vi "onStart.vi"(8 "error in (no error)":errorcluster, 11 "DAQmx":refnum<class "DAQmx.lvclass">) -> (0 "error out":errorcluster, 3 "DAQmx out":refnum<class "DAQmx.lvclass">)   [LabVIEW 2016, in "DAQmx.lvclass"]
doc: "JKI State Machine Objects (SMO) 1.2.1.55\nJKI - JKI\nCopyright (c) 2017, JKI"
uses:
  DAQmx.lvclass
  DAQ/DAQ.lvclass
panel:
  # "For instructions on how to use the JKI State Machine Objects, examples and video tutorials, visit:\nhttp://jki.net/state-machine-objects/\n\nJKI State Machine Objects™\nhttp://jki.net/state-machine-objects/\nCopyright (C) 2005-2015, JKI <info@jki.net>\nALL RIGHTS RESERVED"
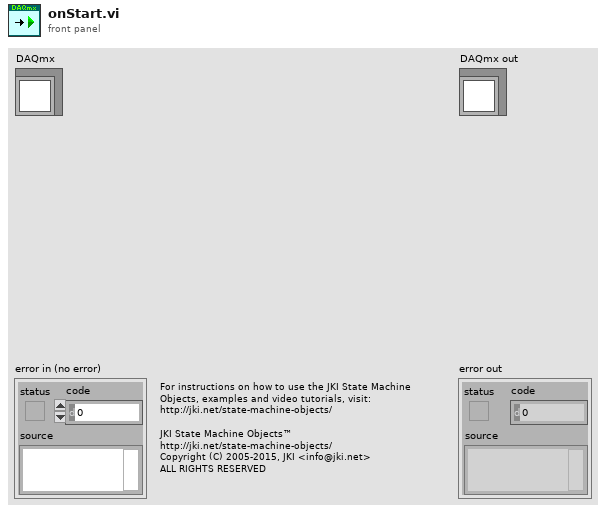
[diagram p1: front panel]
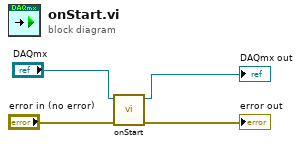
[diagram p0: block diagram]
diagram:
  n1 = call-parent "onStart.vi"("error in (no error)"="error in (no error)", "DAQ"="DAQmx") -> ("error out"=→"error out":errorcluster, "DAQ out"=→"DAQmx out":refnum<class "DAQmx.lvclass">)  [unwired: 8 in]
